vi "build token URI.vi"(8 "error in (no error)":errorcluster, 11 "Oauth2.Google in":refnum<class "Oauth2.Google.lvclass">) -> (0 "error out":errorcluster, 1 "Headers":cluster{"header":string, "value":string}[](array[cluster]), 2 "Token Request URI":string, 3 "Oauth2.Google":refnum<class "Oauth2.Google.lvclass">)   [LabVIEW 2020, in "Oauth2.Google.lvclass"]
uses:
  Oauth2.Google.lvclass
  C:/Data/1_Projects/CIGH_Oauth2/source/Oauth2/Oauth2.lvclass
  Oauth2.Google.lvclass/Oauth2.Google.ctl
  <vilib>/LabVIEW Open Source Project/OpenURI/uri/URI.lvclass
  OAuthToken/OAuth2 Token Element -- enum.ctl
  OAuthToken/OAuthAccessToken.lvclass
  Oauth2/Oauth2.lvclass
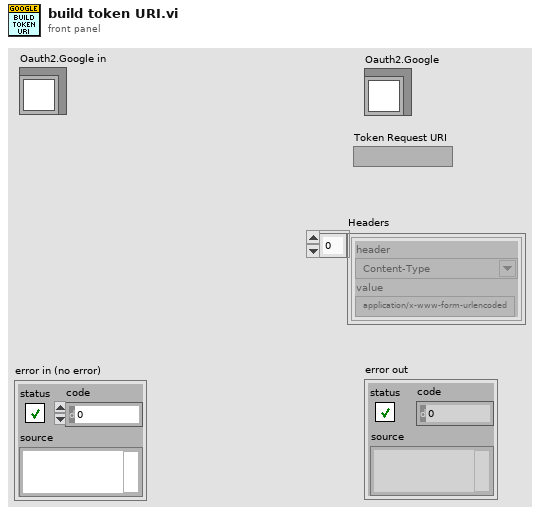
[diagram p1: front panel]
types:
  T1 = typedef "OAuthAccessToken.lvclass/OAuth2 Token Element -- enum.ctl" = enum16{"client_id", "client_secret", "response_type", "scope", "redirect_uri", "error", "error_description", "error_uri", "grant_type", "code", "access_token", "token_type", "expires_in", "username", "password", "refresh_token", "code_challenge", "code_challenge_method", "reverse_proxy_uri", "endpoint element"}
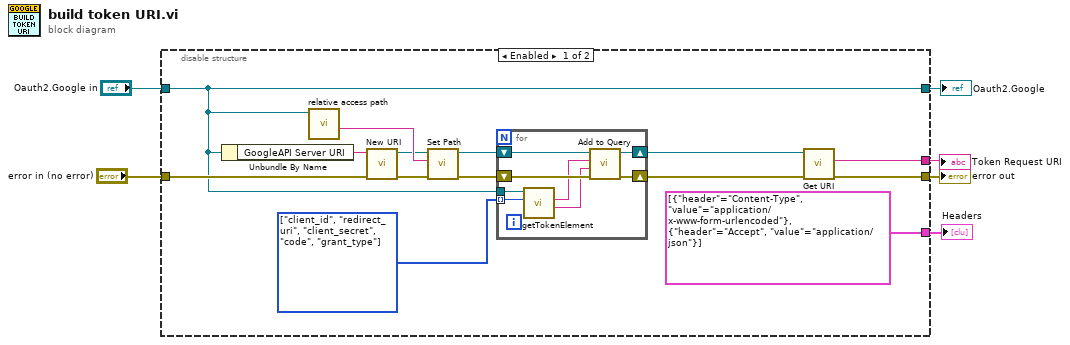
[diagram p0: block diagram]
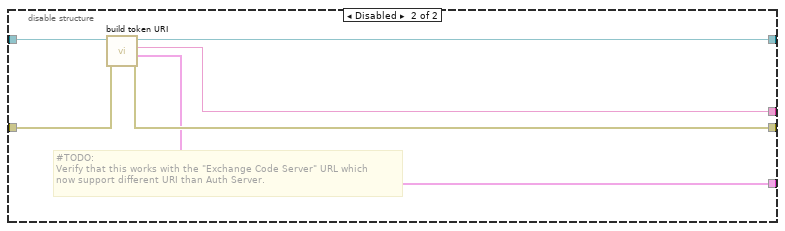
[diagram p2: hidden frame]
diagram:
  n1 = disable-structure shown="Enabled" {
    disable-tunnel: [w13 w32] -> w6
    disable-tunnel: "Oauth2.Google in" -> [w8 w34]
    disable-tunnel: [w11 w30] -> w4
    disable-tunnel: "error in (no error)" -> [w10 w31]
    disable-tunnel: [w8 w33] -> w2
    disable-tunnel: [cluster{"header":string, "value":string}[] [{"header"="Content-Type", "value"="application/x-www-form-urlencoded"}, {"header"="Accept", "value"="application/json"}] ("Headers") w29] -> w1
    frame Enabled {
      w12 = T1[] [enum."client_id", enum."redirect_uri", enum."client_secret", enum."code", enum."grant_type"] items=["client_id", "client_secret", "response_type", "scope", "redirect_uri", "error", "error_description", "error_uri", "grant_type", "code", "access_token", "token_type", "expires_in", "username", "password", "refresh_token", "code_challenge", "code_challenge_method", "reverse_proxy_uri", "endpoint element"]
      n2 = Unbundle By Name(w8) -> ("GoogleAPI Server URI"=w15:string)
      n3 = call-dynamic "relative access path.vi"("Oauth2.Google"=w8) -> ("Token Access Path"=w20:string)  [unwired: 9 in, 1 out]
      n4 = call <vilib>:"New URI.vi"("error in (no error)"=w10, "URI"=w15) -> ("error out"=w9:errorcluster, "URI"=w14:refnum<class "URI.lvclass">)  [unwired: 8 in]
      n5 = call <vilib>:"Set Path.vi"("error in (no error)"=w9, "path"=w20, "URI in"=w14) -> ("error out"=w16:errorcluster, "URI out"=w19:refnum<class "URI.lvclass">)  [unwired: 7 in]
      n6 = for {
        shift-right: [w27] -> w18
        shift-left: w19 -> [w28]
        shift-right: [w25] -> w17
        shift-left: w16 -> [w26]
        tunnel: w8 -> [w24]
        tunnel: w12 -> [w21] mode=indexing
        n7 = call "getTokenElement.vi"("Token element"=w21, "Oauth2 in"=w24) -> ("Value"=w22:string, "Key"=w23:string)  [unwired: 5 in, 3 out]
        n8 = call <vilib>:"Add to Query.vi"("error in (no error)"=w26, "value"=w22, "key"=w23, "URI in"=w28) -> ("error out"=w25:errorcluster, "URI out"=w27:refnum<class "URI.lvclass">)  [unwired: 6 in]
      }
      n9 = call <vilib>:"Get URI.vi"("error in (no error)"=w17, "URI in"=w18) -> ("error out"=w11:errorcluster, "URI String"=w13:string)  [unwired: 7 in, 1 out]
    }
    frame Disabled {
      # "#TODO: \nVerify that this works with the \"Exchange Code Server\" URL which\nnow support different URI than Auth Server."
      n10 = call-parent "build token URI.vi"("error in (no error)"=w31, "Oauth2 in"=w34) -> ("error out"=w30:errorcluster, "Headers"=w29:cluster{"header":string, "value":string}[], "Token Request URI"=w32:string, "Oauth2"=w33:refnum<class "Oauth2.Google.lvclass">)  [unwired: 6 in]
    }
  }
  "Token Request URI" <- w6
  "Oauth2.Google" <- w2
  "error out" <- w4
  "Headers" <- w1
